vi "ProdaNG.Convert.String-DBL.vi"(11 "unsigned byte string":string) -> (3 "dbl integer":dbl)   [LabVIEW 2016]
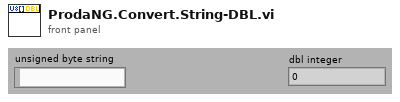
[diagram p1: front panel]
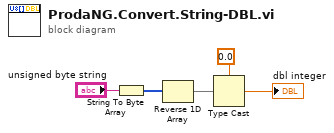
[diagram p0: block diagram]
diagram:
  n1 = String To Byte Array(string="unsigned byte string") -> (unsigned byte array=w4:u8[])
  n2 = Reverse 1D Array(array=w4) -> (reversed array=w1:u8[])
  n3 = Type Cast(type=0.0 ("dbl integer"), x=w1) -> (*(type *) &x=→"dbl integer":dbl)
